vi "Sequence Loop Async.vi"(11 "Tester in":refnum<class "Tester.lvclass">) -> ()   [LabVIEW 2020, in "Tester.lvlib" / "Tester.lvclass"]
uses:
  Tester.lvclass
  Tester.lvclass/Tester.ctl
  Sequence/Sequence.lvclass
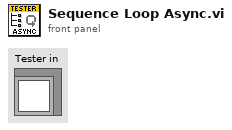
[diagram p1: front panel]
types:
  T1 = typedef "Tester.lvlib/Tester.lvclass/Execution Ref.ctl" = cluster{"Sequence":refnum<class "Sequence.lvclass">, "Step":i32, "Results":refnum<class "Results.lvclass">, "State":T2, "Run Step VI":refnum<vi>, "Abort":bool}
  T2 = typedef "Tester.lvlib/Tester.lvclass/State.ctl" = enum16{"Idle", "In Progress", "Completed"}
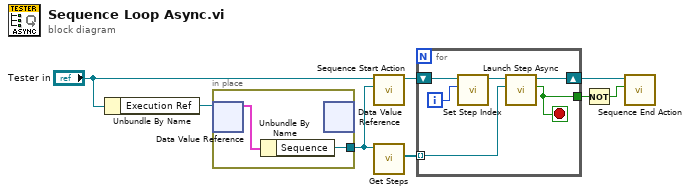
[diagram p0: block diagram]
diagram:
  n1 = Unbundle By Name("Tester in") -> ("Execution Ref"=w8:refnum<data-value>)
  n2 = in-place {
    in-place-border: [w9] -> w6
    n3 = in-place-dvr #1(w8) -> (w10:T1)  [unwired: 1 out]
    n4 = Unbundle By Name(w10) -> ("Sequence"=w9:refnum<class "Sequence.lvclass">)
    n5 = in-place-dvr #1() -> ()  [unwired: 1 in, 2 out]
  }
  n6 = call-dynamic "Sequence Start Action.vi"("Sequence"=w6, "Tester in"="Tester in") -> ("Tester out"=w5:refnum<class "Tester.lvclass">)  [unwired: 8 in, 1 out]
  n7 = call "Get Steps.vi"("Sequence in"=w6) -> ("Steps"=w4:refnum<class "Step.lvclass">[])  [unwired: 8 in, 2 out]
  n8 = for {
    shift-right: [w14] -> w3
    shift-left: w5 -> [w16]
    tunnel: w4 -> [w11] mode=indexing
    tunnel: [w13] -> w2
    i -> [w15]
    stop <- w13 stop-if-true
    n9 = call "Set Step Index.vi"("Step Index"=w15, "Tester in"=w16) -> ("Tester out"=w12:refnum<class "Tester.lvclass">)  [unwired: 8 in, 1 out]
    n10 = call "Launch Step Async.vi"("Step in"=w11, "Tester in"=w12) -> ("Terminate"=w13:bool, "Tester out"=w14:refnum<class "Tester.lvclass">)  [unwired: 7 in, 1 out]
  }
  n11 = Not(x=w2) -> (.not. x?=w1:bool)
  n12 = call-dynamic "Sequence End Action.vi"("Complete"=w1, "Tester in"=w3) -> ()  [unwired: 8 in, 2 out]
